vi "sub_lidar-data_to_vision-data.vi"(11 "img-data2d in":u8[][](array[numeric])) -> (3 "img-data2d out":u8[][](array[numeric]))   [LabVIEW 2019]
uses:
  Ctrl/vlp-16 cmd.ctl
  Ctrl/tim571-databuf.ctl
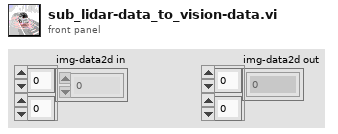
[diagram p1: front panel]
types:
  T1 = typedef "tim571-databuf.ctl" = enum16{"write raw data", "write xyz data", "read"}
  T2 = typedef "vlp-16 cmd.ctl" = enum16{"write all data", "write xyz data", "read"}
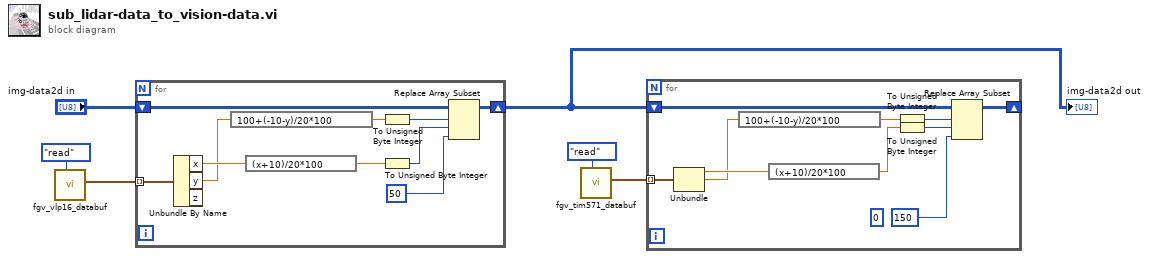
[diagram p0: block diagram]
diagram:
  n1 = call "fgv_vlp16_databuf.vi"("cmd"=vlp-16_cmd."read") -> ("xyz_data_out"=w5:cluster{"x":dbl, "y":dbl, "z":dbl}[])  [unwired: 8 in, 2 out]
  n2 = for {
    tunnel: w5 -> [w16] mode=indexing
    shift-right: [w10] -> w1
    shift-left: "img-data2d in" -> [w11]
    n3 = Unbundle By Name(w16) -> ("x"=w13:dbl, "y"=w12:dbl)  [unwired: 1 out]
    n4 = expression code="100+(-10-y)/20*100"(w12) -> (w14:dbl)
    n5 = expression code="(x+10)/20*100"(w13) -> (w15:dbl)
    n6 = To Unsigned Byte Integer(number=w14) -> (unsigned 8bit integer=w9:u8)
    n7 = To Unsigned Byte Integer(number=w15) -> (unsigned 8bit integer=w8:u8)
    n8 = Replace Array Subset(array=w11, new element=u8 50 ("new element/subarray"), index (row)=w9, index (col)=w8) -> (w10:u8[][])
  }
  "img-data2d out" <- w1
  n9 = call "fgv_tim571_databuf.vi"("cmd"=tim571-databuf."read") -> ("XYZ_DATA out"=w4:cluster{"x":sgl, "y":sgl, "Z":sgl}[])  [unwired: 8 in, 2 out]
  n10 = for {
    tunnel: w4 -> [w26] mode=indexing
    shift-right: [w19] -> _
    shift-left: w1 -> [w20]
    (unwired) u8 0 ("new element/subarray")
    n11 = Unbundle(w26) -> ("x"=w18:sgl, "y"=w17:sgl)  [unwired: 1 out]
    n12 = expression code="100+(-10-y)/20*100"(w17) -> (w24:sgl)
    n13 = expression code="(x+10)/20*100"(w18) -> (w25:sgl)
    n14 = To Unsigned Byte Integer(number=w24) -> (unsigned 8bit integer=w23:u8)
    n15 = To Unsigned Byte Integer(number=w25) -> (unsigned 8bit integer=w22:u8)
    n16 = Replace Array Subset(array=w20, new element=u8 150 ("new element/subarray"), index (row)=w23, index (col)=w22) -> (w19:u8[][])
  }
